vi "Initialize.vi"(8 "error in":errorcluster, 11 "shared resources in":refnum<class "Shared Resources.lvclass">) -> (0 "error out":errorcluster, 3 "shared resources out":refnum<class "Shared Resources.lvclass">)   [LabVIEW 2024, in "AIM ARINC 429 Engine.lvlib" / "Interfaces.lvlib" / "Shared Resources.lvclass"]
uses:
  Shared Resources.lvclass
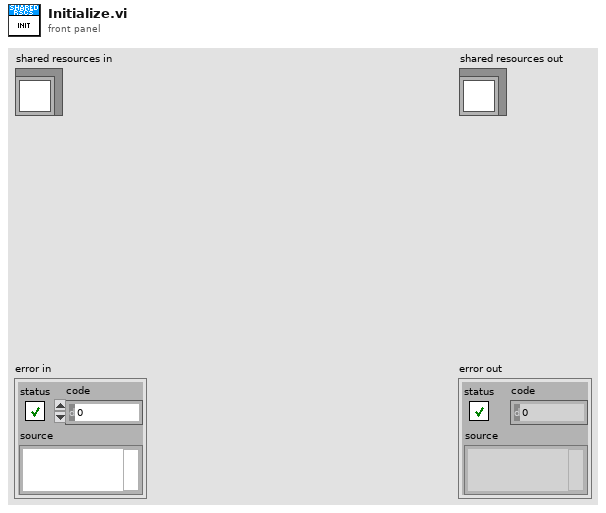
[diagram p1: front panel]
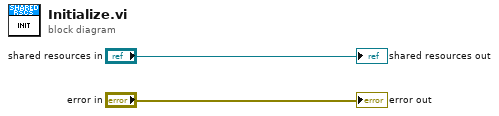
[diagram p0: block diagram]
diagram:
  "error out" <- "error in"
  "shared resources out" <- "shared resources in"
